vi "NtfyLvFpga_SUB_SendMail.vi"(4 "Body":string, 6 "Subject":string, 8 "error in (no error)":errorcluster caption="エラー入力（エラーなし）", 10 "SendTo":T1, 11 "SMTP Setting":T2={"smtp server"="", "From"="", "port number"=25, "userID"="", "password"="", "chk ssl"=FALSE, "chk server withSSL"=FALSE}) -> (0 "error out":errorcluster caption="エラー出力")   [LabVIEW 2013]
uses:
  NtfyLvFpga_Typedef_SMTPSetting.ctl
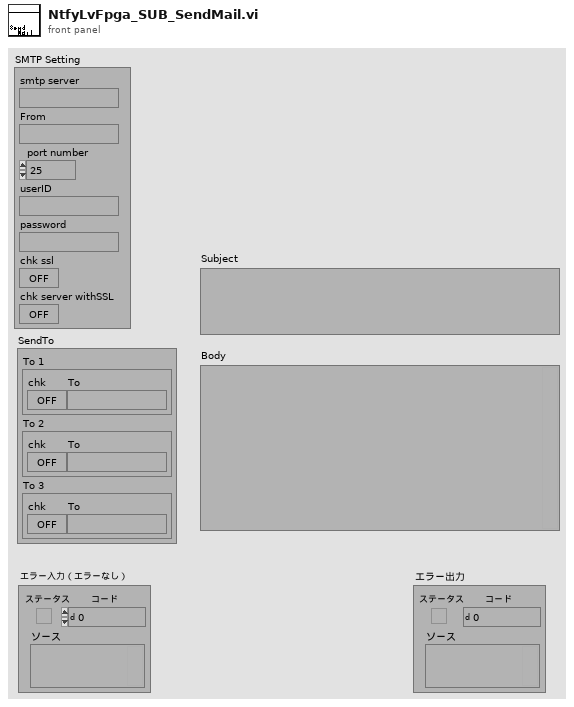
[diagram p1: front panel]
types:
  T1 = cluster{"To 1":cluster{"chk":bool, "To":string}, "To 2":cluster{"chk":bool, "To":string}, "To 3":cluster{"chk":bool, "To":string}}
  T2 = typedef "NtfyLvFpga_Typedef_SMTPSetting.ctl" = cluster{"smtp server":string, "From":string, "port number":i32, "userID":string, "password":string, "chk ssl":bool, "chk server withSSL":bool}
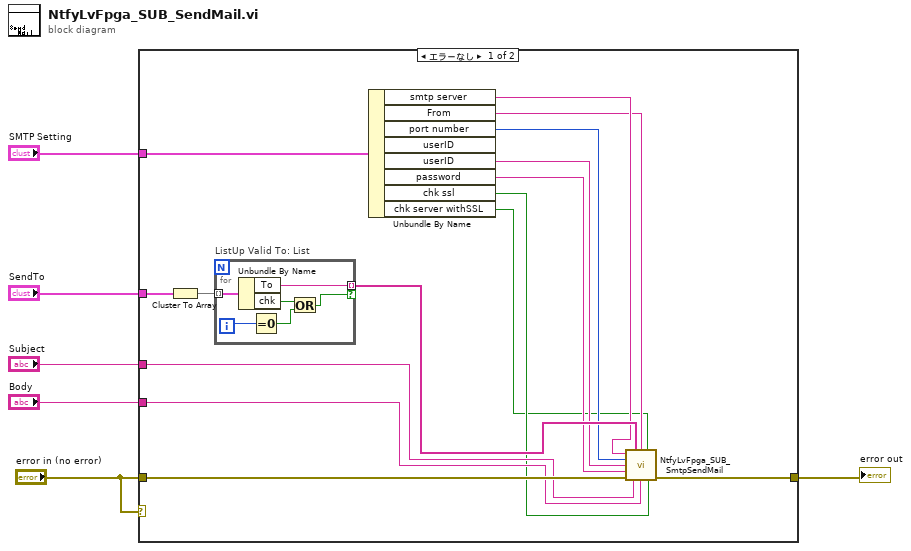
[diagram p0: block diagram]
diagram:
  n1 = case shown="エラーなし" "error in (no error)" {
    tunnel: "error in (no error)" -> [w19 w28]
    tunnel: [w18 w28] -> w5
    tunnel: "SendTo" -> [w21 _]
    tunnel: "SMTP Setting" -> [w16 _]
    tunnel: "Subject" -> [w13 _]
    tunnel: "Body" -> [w12 _]
    frame No Error {
      n2 = Cluster To Array(cluster=w21) -> (array=w20:cluster{"chk":bool, "To":string}[])
      n3 = for "ListUp Valid To: List" {
        tunnel: w20 -> [w26] mode=indexing
        tunnel: [w23] -> w17 mode=indexing if=w22
        i -> [w27]
        n4 = Unbundle By Name(w26) -> ("To"=w23:string, "chk"=w25:bool)
        n5 = Equal To 0?(x=w27) -> (x = 0?=w24:bool)
        n6 = Or(x=w25, y=w24) -> (x .or. y?=w22:bool)
      }
      n7 = Unbundle By Name(w16) -> ("smtp server"=w15:string, "From"=w14:string, "port number"=w11:i32, "userID"=w10:string, "password"=w9:string, "chk ssl"=w8:bool, "chk server withSSL"=w7:bool)  [unwired: 1 out]
      n8 = call "NtfyLvFpga_SUB_SmtpSendMail.vi"("smtp server"=w15, "to[]"=w17, "from"=w14, "Chk Server withSSL"=w7, "portNo(25)"=w11, "User-Id"=w10, "password"=w9, "error in (no error)"=w19, "subject"=w13, "body"=w12, "SSL"=w8) -> ("error out"=w18:errorcluster)  [unwired: 4 in]
    }
    frame Error {
    }
  }
  "error out" <- w5
